vi "PDP Send User Comment.vi"(0 "?":string) -> ()   [LabVIEW 2019]
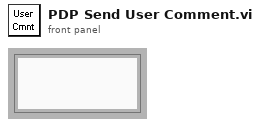
[diagram p1: front panel]
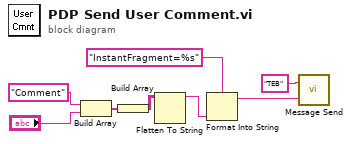
[diagram p0: block diagram]
diagram:
  n1 = Build Array("Comment", "?") -> (w6:string[])
  n2 = Build Array(w6) -> (w1:string[][])
  n3 = Flatten To String(anything=w1) -> (data string=w3:string)  [unwired: 3 in, 2 out]
  n4 = Format Into String(format string="InstantFragment=%s" ("Format String"), w3) -> (resulting string=w2:string)  [unwired: 2 in, 1 out]
  n5 = call "Message Send.vi"("Message"=w2, "Destination"="TEB") -> ()
